vi "Colour Processing Test Env.vi"() -> (0 "Colour scan time out?":bool, 3 "Colour output boolean cluster":T1)   [LabVIEW 2018]
uses:
  Underlying VI's/Modified webcam FGV/Webcam AE.ctl
  <vilib>/userdefined/High Color/IMAQdx.ctl
  Underlying VI's/I2C Master VI/Arduino_Interfacing.ctl
  Underlying VI's/I2C Master VI/I2C_MASTER_WRITE_NEW Type Def.ctl
  Underlying VI's/Elasped Timer/Elapsed timer control.ctl
panel:
  out "Position reached?":bool
  out "Time Out?!":bool
  out "Arduino Data":T2
  out "error out":errorcluster
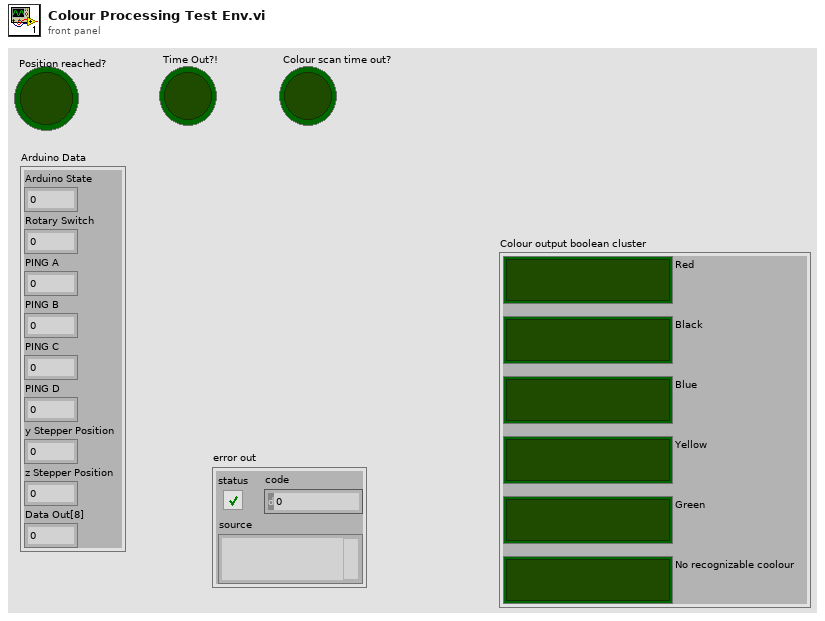
[diagram p1: front panel]
types:
  T1 = cluster{"Red":bool, "Black":bool, "Blue":bool, "Yellow":bool, "Green":bool, "No recognizable coolour":bool}
  T2 = cluster{"Arduino State":u8, "Rotary Switch":u8, "PING A":u8, "PING B":u8, "PING C":u8, "PING D":u8, "y Stepper Position":u8, "z Stepper Position":u8, "Data Out[8]":u8}
  T3 = typedef "Webcam AE.ctl" = enum16{"Initialize Camera", "Open Camera", "Continuous Acquisition", "Close Camera", "Retrieve Image", "Dispose Camera Image Buffer"}
  T4 = typedef "IMAQdx.ctl" = refnum<k21>
  T5 = typedef "I2C_MASTER_WRITE_NEW Type Def.ctl" = enum16{"Ultrasonic sensors", "Stepper origin", "zStepper 13.3k", "zStepper 13k", "zStepper 12k", "zStepper 11k", "zStepper 10k", "zStepper 9k", "zStepper 8k", "zStepper 7k", "zStepper 6k", "zStepper 5k", "zStepper 4k", "zStepper 3k", "zStepper 2k", "zStepper 1k", "zStepper 900", "zStepper 800", "zStepper 700", "zStepper 600", "zStepper 500", "zStepper 400", "zStepper 300", "zStepper 200", "zStepper 100", "zStepper 0", "yStepper control", "Open Claw", "Close Claw", "Soft Reset"}
  T6 = typedef "Arduino_Interfacing.ctl" = enum16{"Initialize", "Write to Arduino", "Read From Arduino"}
  T7 = typedef "Elapsed timer control.ctl" = enum16{"Start", "Pause", "Initialize"}
  T8 = typedef "IMAQ Image.ctl" = refnum<image>
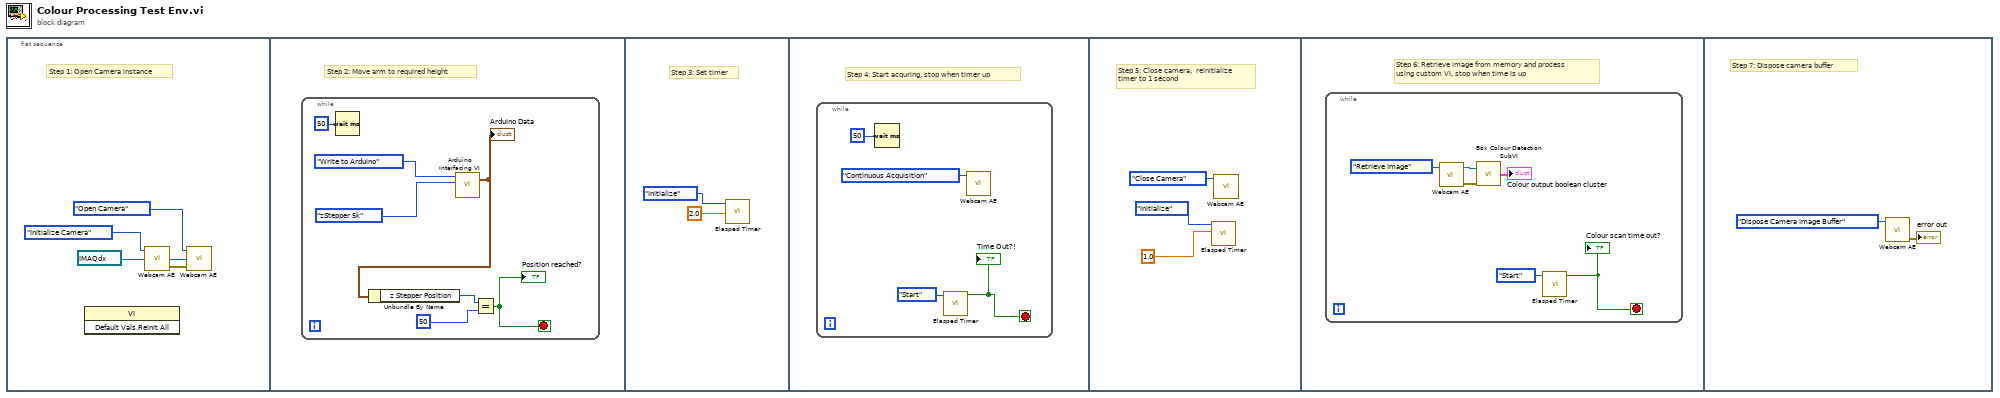
[diagram p0: block diagram]
diagram:
  n1 = flat-sequence {
    frame #0 {
      # "Step 1: Open Camera instance"
      n2 = invoke class="VI" method="Default Vals.Reinit All"() -> ()  [unwired: 3 in, 3 out]
      n3 = call "Webcam AE.vi"("Session In"=T4 "cam1", "Camera states"=Webcam_AE."Initialize Camera") -> ("error out"=w4:errorcluster, "Session Out"=w5:T4)  [unwired: 1 in, 1 out]
      n4 = call "Webcam AE.vi"("error in (no error)"=w4, "Session In"=w5, "Camera states"=Webcam_AE."Open Camera") -> ()  [unwired: 3 out]
    }
    frame #1 {
      # "Step 2: Move arm to required height"
      n5 = while {
        stop <- w7 stop-if-true
        n6 = Wait (ms)(milliseconds to wait=u32 50) -> ()  [unwired: 1 out]
        n7 = call "Arduino Interfacing VI.vi"("Data to Write"=I2C_MASTER_WRITE_NEW_Type_Def."zStepper 5k", "AE Mode"=Arduino_Interfacing."Write to Arduino") -> ("Arduino Data"=w9:T2)  [unwired: 2 in, 1 out]
        "Arduino Data" <- w9
        n8 = Unbundle By Name(w9) -> ("z Stepper Position"=w6:u8)
        n9 = Equal?(x=w6, y=u8 50) -> (x = y?=w7:bool)
        "Position reached?" <- w7
      }
    }
    frame #2 {
      # "Step 3: Set timer"
      n10 = call "Elasped Timer.vi"("Time Setting"=2.0, "Action"=Elapsed_timer_control."Initialize") -> ()  [unwired: 6 in, 4 out]
    }
    frame #3 {
      # "Step 4: Start acquring, stop when timer up"
      n11 = while {
        stop <- w15 stop-if-true
        n12 = Wait (ms)(milliseconds to wait=u32 50 ("millisecond timer value")) -> ()  [unwired: 1 out]
        n13 = call "Elasped Timer.vi"("Action"=Elapsed_timer_control."Start") -> ("Time Out?!"=w15:bool)  [unwired: 7 in, 3 out]
        "Time Out?!" <- w15
        n14 = call "Webcam AE.vi"("Camera states"=Webcam_AE."Continuous Acquisition") -> ()  [unwired: 2 in, 3 out]
      }
    }
    frame #4 {
      # "Step 5: Close camera,  reinitialize \ntimer to 1 second"
      n15 = call "Elasped Timer.vi"("Time Setting"=1.0, "Action"=Elapsed_timer_control."Initialize") -> ()  [unwired: 6 in, 4 out]
      n16 = call "Webcam AE.vi"("Camera states"=Webcam_AE."Close Camera") -> ()  [unwired: 2 in, 3 out]
    }
    frame #5 {
      # "Step 6: Retrieve image from memory and process\nusing custom VI, stop when time is up"
      n17 = while {
        stop <- w23 stop-if-true
        n18 = call "Webcam AE.vi"("Camera states"=Webcam_AE."Retrieve Image") -> ("error out"=w25:errorcluster, "Image Out"=w26:T8)  [unwired: 2 in, 1 out]
        n19 = call "Box Colour Detection SubVI.vi"("Image In"=w26, "Error In"=w25) -> ("Colour output boolean cluster"=→"Colour output boolean cluster":T1)  [unwired: 2 out]
        n20 = call "Elasped Timer.vi"("Action"=Elapsed_timer_control."Start") -> ("Time Out?!"=w23:bool)  [unwired: 7 in, 3 out]
        "Colour scan time out?" <- w23
      }
    }
    frame #6 {
      # "Step 7: Dispose camera buffer"
      n21 = call "Webcam AE.vi"("Camera states"=Webcam_AE."Dispose Camera Image Buffer") -> ("error out"=→"error out":errorcluster)  [unwired: 2 in, 2 out]
    }
  }
